vi "DBCommentsCompile.vi"() -> (0 "Comments out":string)   [LabVIEW 2013]
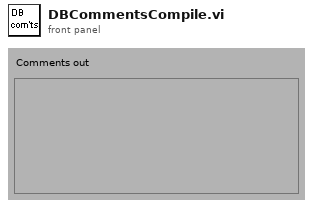
[diagram p1: front panel]
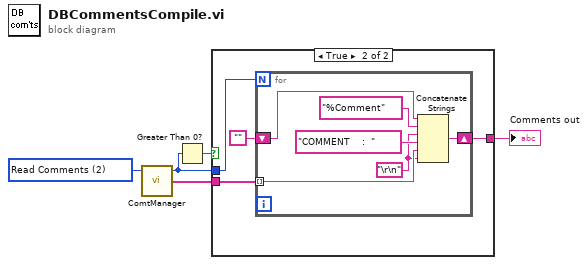
[diagram p0: block diagram]
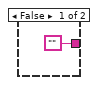
[diagram p2: hidden frame]
diagram:
  w5 = u16 2 items=["Initialise", "Add comment", "Read Comments"] ("Action")
  n1 = call "ComtManager.vi"("Action"=w5) -> ("Comments out"=w4:string[], "No of comments"=w2:i32)  [unwired: 2 in, 1 out]
  n2 = Greater Than 0?(x=w2) -> (x > 0?=w1:bool)
  n3 = case shown="True" w1 {
    tunnel: w2 -> [_ w10]
    tunnel: w4 -> [_ w9]
    tunnel: ["" w7] -> w3
    frame False {
    }
    frame True {
      n4 = for {
        N: w10 -> [_]
        tunnel: w9 -> [w12] mode=indexing
        shift-right: [w14] -> w7
        shift-left: "" -> [w16]
        w11 = "\r\n"
        n5 = Concatenate Strings(w16, "%Comment", w11, "COMMENT    :  ", w12, w11) -> (w14:string)
      }
    }
  }
  "Comments out" <- w3
